vi "DoOperationStaticDispatchMethod - Reentrant.vi"(8 "error in (no error)":errorcluster, 11 "SimpleArithmetic in":refnum<class "SimpleArithmetic - Reentrant.lvclass">) -> (0 "error out":errorcluster, 3 "SimpleArithmetic out":refnum<class "SimpleArithmetic - Reentrant.lvclass">)   [LabVIEW 2010, in "SimpleArithmetic - Reentrant.lvclass"]
uses:
  SimpleArithmetic - Reentrant.lvclass
  SimpleArithmetic - Reentrant.lvclass/SimpleArithmetic - Reentrant.ctl
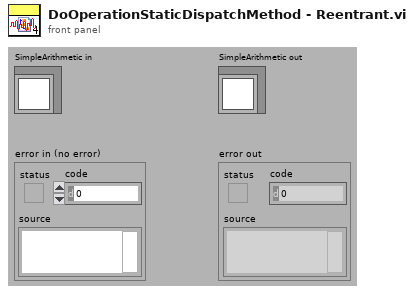
[diagram p1: front panel]
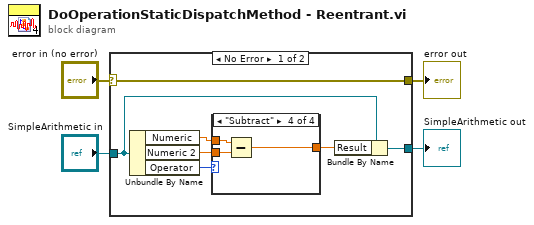
[diagram p0: block diagram]
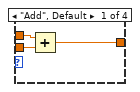
[diagram p2: hidden frame]
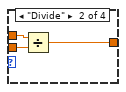
[diagram p3: hidden frame]
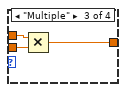
[diagram p4: hidden frame]
diagram:
  n1 = case shown="No Error" "error in (no error)" {
    selector: "error in (no error)" -> [w11 w25]
    tunnel: [w11 w25] -> w3
    tunnel: [w8 w24] -> w1
    tunnel: "SimpleArithmetic in" -> [w9 w24]
    frame No Error {
      n2 = Unbundle By Name(w9) -> ("Numeric"=w7:dbl, "Numeric 2"=w6:dbl, "Operator"=w10:enum16{"Add", "Divide", "Multiple", "Subtract"})
      n3 = case shown="\"Subtract\"" w10 {
        tunnel: w7 -> [w14 w17 w20 w23]
        tunnel: w6 -> [w13 w16 w19 w22]
        tunnel: [w12 w15 w18 w21] -> w5
        frame "Add", Default {
          n4 = Add(x=w14, y=w13) -> (x+y=w12:dbl)
        }
        frame "Divide" {
          n5 = Divide(x=w17, y=w16) -> (x/y=w15:dbl)
        }
        frame "Multiple" {
          n6 = Multiply(x=w20, y=w19) -> (x*y=w18:dbl)
        }
        frame "Subtract" {
          n7 = Subtract(x=w23, y=w22) -> (x-y=w21:dbl)
        }
      }
      n8 = Bundle By Name(cluster=w9, "Result"=w5) -> (w8:refnum<class "SimpleArithmetic - Reentrant.lvclass">)
    }
    frame Error {
    }
  }
  "error out" <- w3
  "SimpleArithmetic out" <- w1
